vi "Data_Array_Initialize.vi"(8 "error in (no error)":errorcluster, 10 "Buffer":i32, 11 "Data_Array in":refnum<class "Data_Array.lvclass">) -> (0 "error out":errorcluster, 3 "Data_Array out":refnum<class "Data_Array.lvclass">)   [LabVIEW 2021, in "Data_Array.lvclass"]
uses:
  Data_Array.lvclass
  Data_Array.lvclass/Data_Array.ctl
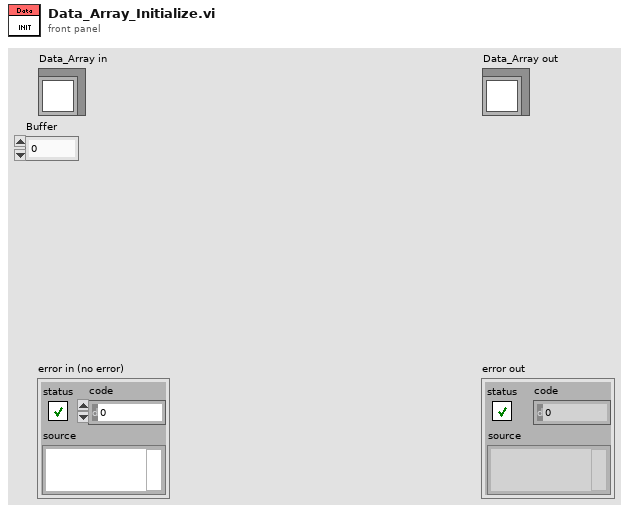
[diagram p1: front panel]
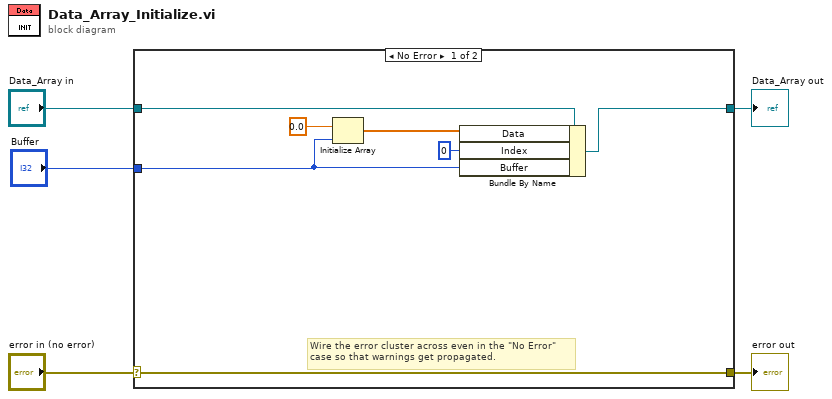
[diagram p0: block diagram]
diagram:
  n1 = case shown="No Error" "error in (no error)" {
    selector: "error in (no error)" -> [w12 w14]
    tunnel: [w12 w14] -> w4
    tunnel: [w9 w13] -> w2
    tunnel: "Data_Array in" -> [w10 w13]
    tunnel: "Buffer" -> [w7 _]
    frame No Error {
      # "Wire the error cluster across even in the \"No Error\"\ncase so that warnings get propagated."
      n2 = Initialize Array(0.0 ("element"), w7) -> (w8:dbl[])
      n3 = Bundle By Name(cluster=w10, "Data"=w8, "Index"=0 ("Data_params.Index"), "Buffer"=w7) -> (w9:refnum<class "Data_Array.lvclass">)
    }
    frame Error {
    }
  }
  "error out" <- w4
  "Data_Array out" <- w2
